vi "action.vi"(0 "HGF_SVVarManVisitor_delete":refnum<class "HGF_SVVarManVisitor_delete.lvclass">, 2 "HGF_Visitable":refnum<class "HGF_Visitable.lvclass">, 5 "error in (no error)":errorcluster) -> (14 "dup HGF_SVVarManVisitor_delete":refnum<class "HGF_SVVarManVisitor_delete.lvclass">, 16 "dup HGF_Visitable":refnum<class "HGF_Visitable.lvclass">, 19 "error out":errorcluster)   [LabVIEW 2012, in "HGF_SV.lvlib" / "HGF_SVVarManVisitor_delete.lvclass"]
doc: "This is a dynamic dispatch VI that is called from Visitor.visit(). It will call member VIs of Visitable to perform the requested action which means: calling public methods of Visitable child class.\n\n<B>Hint:</B> This method is abstract and need to be implemented by child classes."
uses:
  HGF_SVVarManVisitor_delete.lvclass
  HGF_BaseClasses/HGF_Visitable/HGF_Visitable.lvclass
  HGF_DSC/HGF_DSCVarManager/HGF_DSCVarManager.lvclass
  HGF_BaseClasses/HGF_Visitor/HGF_Visitor.lvclass
  HGF_SVVarManVisitor_delete.lvclass/HGF_SVVarManVisitor_delete.ctl
  HGF_BaseClasses/HGF_TriggeredEvent/HGF_TriggeredEvent.lvclass
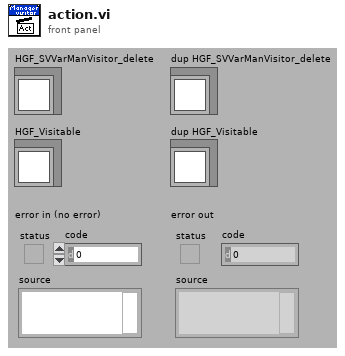
[diagram p1: front panel]
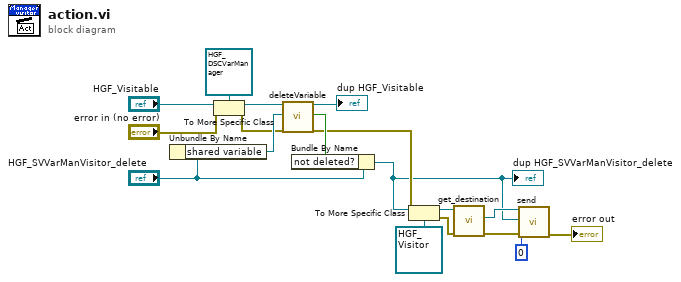
[diagram p0: block diagram]
diagram:
  n1 = Unbundle By Name("HGF_SVVarManVisitor_delete") -> ("shared variable"=w14:refnum<k21>)
  n2 = To More Specific Class(target class=refnum<class "HGF_DSCVarManager.lvclass"> refnum ("DSC.lvlib:HGF_DSCVarManager.lvclass"), reference="HGF_Visitable", error in="error in (no error)") -> (specific class reference=w16:refnum<class "HGF_DSCVarManager.lvclass">, error out=w2:errorcluster)
  n3 = call-dynamic "deleteVariable.vi"("HGF_DSCVarManager in"=w16, "shared variable"=w14, "error in (no error)"=w2) -> ("HGF_DSCVarManager out"=→"dup HGF_Visitable":refnum<class "HGF_DSCVarManager.lvclass">, "not deleted?"=w13:bool, "error out"=w9:errorcluster)  [unwired: 14 in]
  n4 = Bundle By Name(cluster="HGF_SVVarManVisitor_delete", "not deleted?"=w13) -> (w5:refnum<class "HGF_SVVarManVisitor_delete.lvclass">)
  "dup HGF_SVVarManVisitor_delete" <- w5
  n5 = To More Specific Class(target class=refnum<class "HGF_Visitor.lvclass"> refnum ("HGF_BaseClasses.lvlib:HGF_Visitor.lvclass"), reference=w5, error in=w9) -> (specific class reference=w10:refnum<class "HGF_Visitor.lvclass">, error out=w8:errorcluster)
  n6 = call "get_destination.vi"("error in (no error)"=w8, "HGF_Visitor"=w10) -> ("error out"=w7:errorcluster, "destination"=w6:refnum<class "HGF_TriggeredEvent.lvclass">)  [unwired: 7 in, 1 out]
  n7 = call-dynamic "send.vi"("HGF_Event"=w6, "Object"=w5, "timeout in ms (-1)"=0, "error in (no error)"=w7) -> ("error out"=→"error out":errorcluster)  [unwired: 13 in, 2 out]
